vi "Set Display Main Page Title.vi"(9 "VI Ref":refnum<vi>, 11 "Stand Alone Display Actor in":refnum<class "Stand Alone Display Actor.lvclass">) -> (3 "Stand Alone Display Actor out":refnum<class "Stand Alone Display Actor.lvclass">)   [LabVIEW 2024, in "Stand Alone Display Actor.lvclass"]
uses:
  Stand Alone Display Actor.lvclass
  Ancestor Class/Actor/System Actor/System Actor.lvclass/System Actor.ctl
  Ancestor Class/Actor/System Actor/Public Data/Read Actor Name.vi
  Stand Alone Display Actor.lvclass/Stand Alone Display Actor.ctl
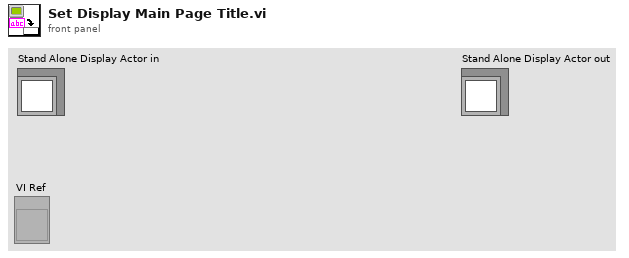
[diagram p1: front panel]
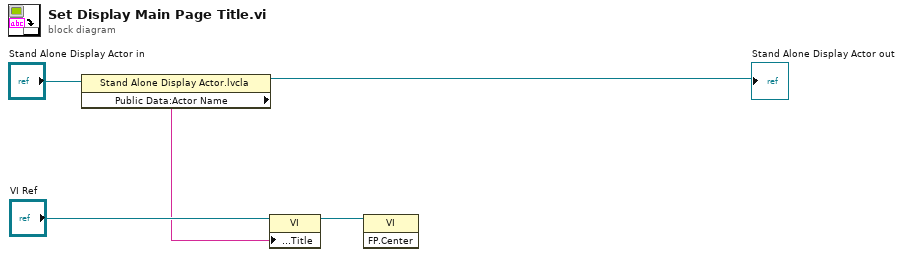
[diagram p0: block diagram]
diagram:
  n1 = property class="Stand Alone Display Actor.lvcla"(reference="Stand Alone Display Actor in") -> (reference out=→"Stand Alone Display Actor out":refnum<class "Stand Alone Display Actor.lvclass">, "Public Data:Actor Name"=w2:string)  [unwired: 1 in, 1 out]
  n2 = property class="VI"(reference="VI Ref", "Front Panel.Title"=w2) -> (reference out=w1:refnum<vi>)  [unwired: 1 in, 1 out]
  n3 = invoke class="VI" method="FP.Center"(reference=w1) -> ()  [unwired: 2 in, 3 out]
